vi "SimpleQueue.vi"() -> ()   [LabVIEW 2011]
panel:
  out "Waveform Graph":dbl[](graph)
  in  "stop":bool
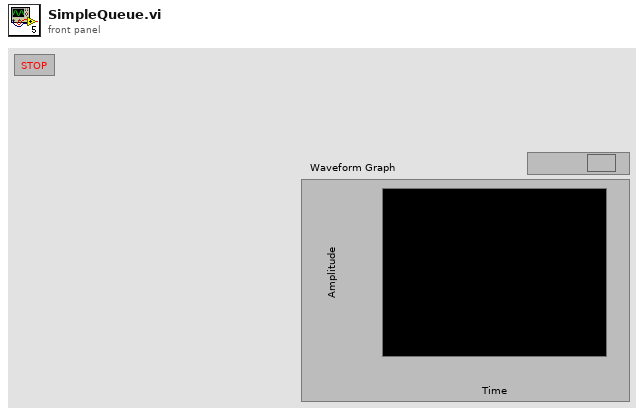
[diagram p1: front panel]
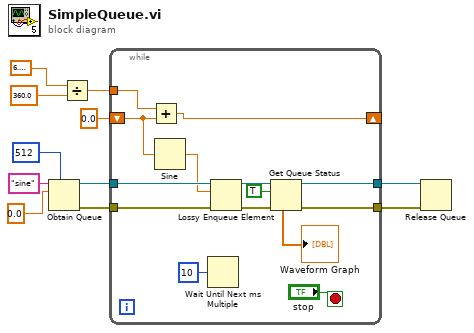
[diagram p0: block diagram]
diagram:
  n1 = Obtain Queue(max queue size (-1, unlimited)=512, name (unnamed)="sine", element data type=0.0) -> (queue out=w8:refnum<queue>, error out=w7:errorcluster)  [unwired: 2 in, 1 out]
  n2 = Divide(x=6.283185307179586, y=360.0) -> (x/y=w4:dbl)
  n3 = while {
    tunnel: w8 -> [w24]
    tunnel: w7 -> [w23]
    tunnel: w4 -> [w22]
    shift-right: [w21] -> _
    shift-left: 0.0 -> [w20]
    tunnel: [w16] -> w2
    tunnel: [w15] -> w1
    stop <- "stop" stop-if-true
    n4 = Add(x=w22, y=w20) -> (x+y=w21:dbl)
    n5 = Sine(x=w20) -> (sin(x)=w19:dbl)
    n6 = Wait Until Next ms Multiple(millisecond multiple=u32 10) -> ()  [unwired: 1 out]
    n7 = Lossy Enqueue Element(queue=w24, element=w19, error in (no error)=w23) -> (queue out=w18:refnum<queue>, error out=w17:errorcluster)  [unwired: 2 out]
    n8 = Get Queue Status(queue=w18, return elements? (F)=TRUE, error in (no error)=w17) -> (queue out=w16:refnum<queue>, error out=w15:errorcluster, elements=→"Waveform Graph":dbl[])  [unwired: 5 out]
  }
  n9 = Release Queue(queue=w2, error in (no error)=w1) -> ()  [unwired: 1 in, 3 out]
